vi "Deinit.vi"(8 "error in (no error)":errorcluster, 11 "IV in":refnum<class "IV.lvclass">) -> (0 "error out":errorcluster, 3 "IV out":refnum<class "IV.lvclass">)   [LabVIEW 2021, in "IV.lvclass"]
uses:
  IV.lvclass
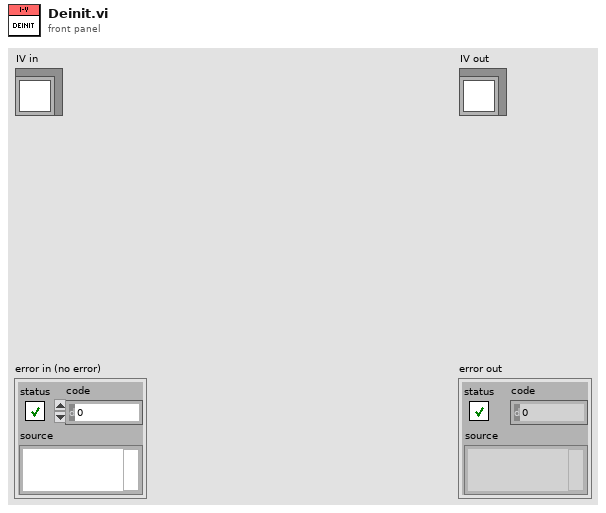
[diagram p1: front panel]
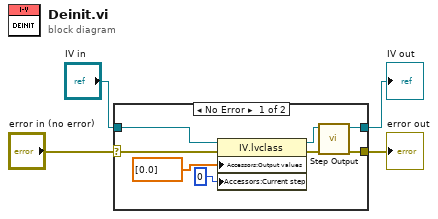
[diagram p0: block diagram]
diagram:
  n1 = case shown="No Error" "error in (no error)" {
    selector: "error in (no error)" -> [w12 w14]
    tunnel: [w5 w14] -> w3
    tunnel: [w7 w13] -> w1
    tunnel: "IV in" -> [w11 w13]
    frame No Error {
      n2 = property class="IV.lvclass"(reference=w11, error in=w12, "Accessors:Output values"=dbl[] [0.0] ("Output values"), "Accessors:Current step"=0 ("Current step")) -> (reference out=w8:refnum<class "IV.lvclass">, error out=w6:errorcluster)
      n3 = call-dynamic "Step Output.vi"("error in (no error)"=w6, "IV in"=w8) -> ("error out"=w5:errorcluster, "IV out"=w7:refnum<class "IV.lvclass">)  [unwired: 8 in]
    }
    frame Error {
    }
  }
  "error out" <- w3
  "IV out" <- w1
